vi "pruebaspy.vi"() -> ()   [LabVIEW 2020]
panel:
  in  "datos":path
  out "return value":string
  out "error out":errorcluster
  in  "programa":path
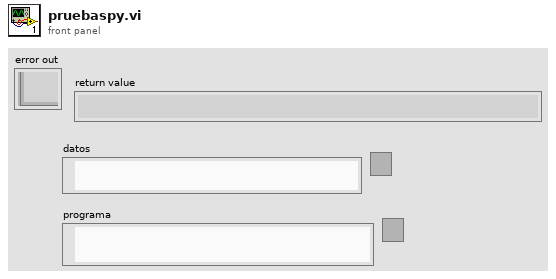
[diagram p1: front panel]
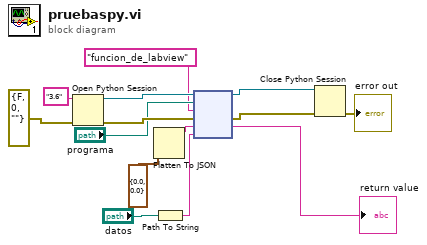
[diagram p0: block diagram]
diagram:
  n1 = Open Python Session(python version="3.6" ("Python version"), 3:errorcluster {"status"=FALSE, "code"=0, "source"=""} ("error in (no error)")) -> (session out=w13:refnum<k35>, error out=w11:errorcluster)  [unwired: 1 in]
  n2 = Flatten To JSON(anything=cluster{dbl, dbl} {0.0, 0.0}) -> (JSON string=w4:string)  [unwired: 2 in, 1 out]
  n3 = Path To String(path="datos") -> (string=w1:string)
  n4 = node(w13, "programa", "funcion_de_labview" ("function name"), w11, w4, w1) -> (w12:refnum<k35>, w6:errorcluster, →"return value":string)  [unwired: 1 in, 2 out]
  n5 = Close Python Session(session in=w12, error in=w6) -> (11:→"error out":errorcluster)
